vi "testWriteFileUtf8EncodingHeaderPresent.vi"(8 "error in (no error)":errorcluster, 11 "TestCase in":refnum<class "EasyXMLTest.lvclass">) -> (0 "error out":errorcluster, 3 "TestCase out":refnum<class "EasyXMLTest.lvclass">)   [LabVIEW 2013, in "EasyXMLTest.lvclass"]
doc: "Verify that no encoding attribute is present if an empty encoding string is specified."
uses:
  EasyXMLTest.lvclass
panel:
  out "XML File Header":string
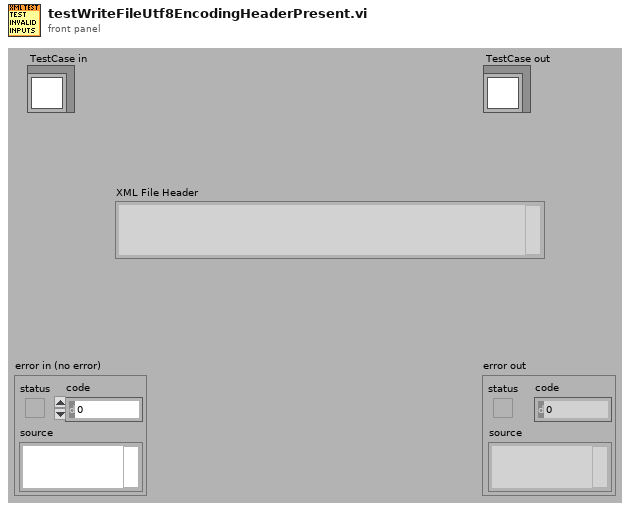
[diagram p1: front panel]
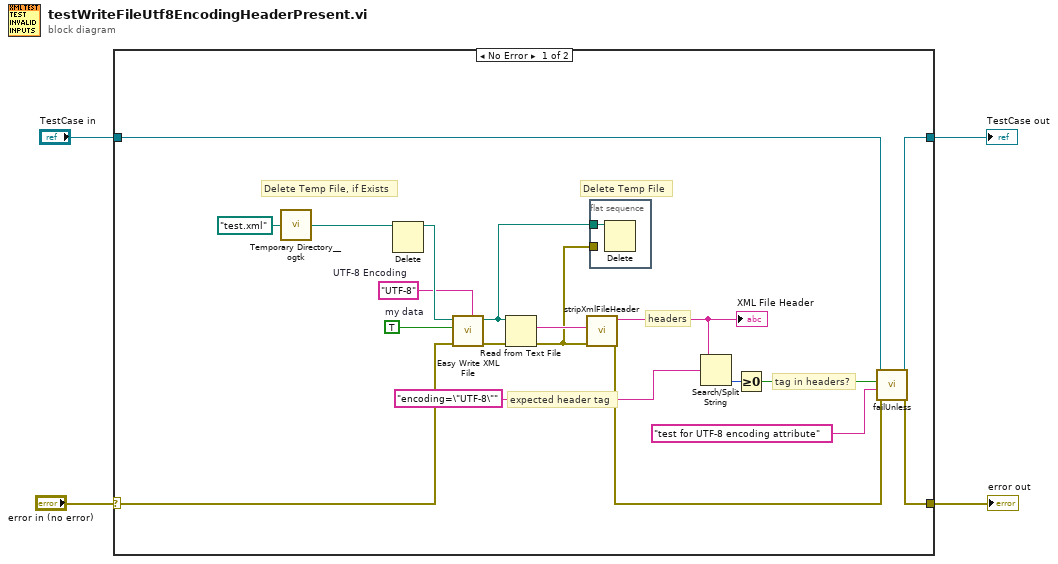
[diagram p0: block diagram]
diagram:
  n1 = case shown="No Error" "error in (no error)" {
    selector: "error in (no error)" -> [w22 w26]
    tunnel: [w9 w26] -> w3
    tunnel: [w11 w25] -> w1
    tunnel: "TestCase in" -> [w12 w25]
    frame No Error {
      w5 = "UTF-8"  # UTF-8 Encoding
      w23 = TRUE  # my data
      # "tag in headers?"
      # "headers"
      # "expected header tag"
      # "Delete Temp File"
      # "Delete Temp File, if Exists"
      n2 = call <userlib>:"Temporary Directory__ogtk.vi"("Relative path (.)"=path "test.xml") -> ("Temporary Directory (+ Relative)"=w20:path)
      n3 = Delete(path (use dialog)=w20) -> (deleted path=w19:path)  [unwired: 4 in, 2 out]
      n4 = call "Easy Write XML File.vi"("Encoding (none)"=w5, "error in (no error)"=w22, "LabVIEW Data"=w23, "XML File Path"=w19) -> ("error out"=w17:errorcluster, "XML File Path (duplicate)"=w18:path)  [unwired: 6 in]
      n5 = Read from Text File(file (use dialog)=w18, error in=w17) -> (text=w16:string, error out=w15:errorcluster)  [unwired: 2 in, 2 out]
      n6 = call "stripXmlFileHeader.vi"("error in (no error)"=w15, "XML File String"=w16) -> ("error out"=w10:errorcluster, "XML File Header"=w14:string)  [unwired: 7 in, 1 out]
      "XML File Header" <- w14
      n7 = flat-sequence {
        tunnel: w18 -> [w24]
        tunnel: w15 -> [_]
        frame #0 {
          n8 = Delete(path (use dialog)=w24) -> ()  [unwired: 4 in, 3 out]
        }
      }
      n9 = Search/Split String(string=w14, search string/char (-)="encoding=\"UTF-8\"") -> (offset of match=w13:i32)  [unwired: 1 in, 2 out]
      n10 = Greater Or Equal To 0?(x=w13) -> (x >= 0?=w8:bool)
      n11 = call-dynamic "failUnless.vi"("error in (no error)"=w10, "message (\"\")"="test for UTF-8 encoding attribute" ("message (\"\")"), "pass"=w8, "TestCase in"=w12) -> ("error out"=w9:errorcluster, "TestCase out"=w11:refnum<class "EasyXMLTest.lvclass">)  [unwired: 6 in]
    }
    frame Error {
    }
  }
  "error out" <- w3
  "TestCase out" <- w1
